vi "Calculate alpha and beta.vi"(3 "Fit parameters":T1, 4 "Frequency (GHz)":dbl) -> (0 "Beta":dbl, 1 "Alpha":dbl)   [LabVIEW 2019]
uses:
  Fit Parameters.ctl
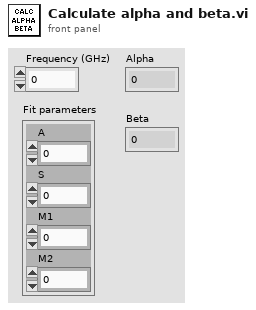
[diagram p1: front panel]
types:
  T1 = typedef "Fit Parameters.ctl" = cluster{"A":dbl, "S":dbl, "M1":dbl, "M2":dbl}
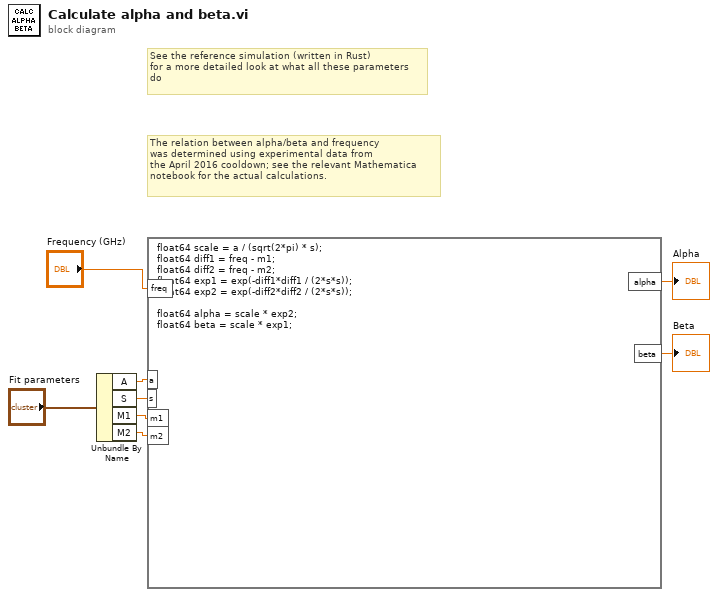
[diagram p0: block diagram]
diagram:
  # "See the reference simulation (written in Rust)\nfor a more detailed look at what all these parameters\ndo"
  # "The relation between alpha/beta and frequency\nwas determined using experimental data from\nthe April 2016 cooldown; see the relevant Mathematica\nnotebook for the actual calculations."
  n1 = Unbundle By Name("Fit parameters") -> ("A"=w4:dbl, "S"=w3:dbl, "M1"=w2:dbl, "M2"=w1:dbl)
  n2 = formula code="float64 scale = a / (sqrt(2*pi) * s);\nfloat64 diff1 = freq - m1;\nfloat64 diff2 = freq - m2;\nfloat64 exp1 = exp(-diff1*diff1 / (2*s*s));\nfloat64 exp2 = exp(-diff2*diff2 / (2*s*s));\n\nfloat64 alpha = scale * exp2;\nfloat64 beta = scale * exp1;"("freq"="Frequency (GHz)", "a"=w4, "s"=w3, "m1"=w2, "m2"=w1) -> ("alpha"=→"Alpha":dbl, "beta"=→"Beta":dbl)
